vi "控件单位.vi"() -> ()   [LabVIEW 2010]
panel:
  out "距离":dbl[unit]
  in  "速度":dbl[unit]
  in  "时间":dbl[unit]
  out "加速度":dbl[unit]
  in  "时间":dbl[unit]
  in  "速度":dbl[unit]
  out "距离":dbl[unit]
  in  "时间":dbl[unit]
  in  "速度":dbl[unit]
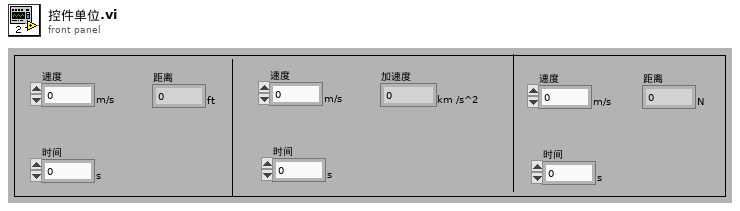
[diagram p1: front panel]
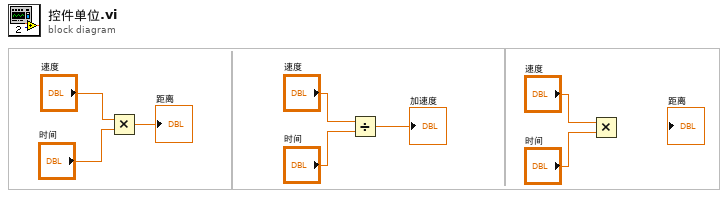
[diagram p0: block diagram]
diagram:
  n1 = Multiply(x="速度", y="时间") -> (x*y=→"距离":dbl[unit])
  n2 = Divide(x="速度", y="时间") -> (x/y=→"加速度":dbl[unit])
  n3 = Multiply(x="速度", y="时间") -> ()  [unwired: 1 out]
